vi "Passing Paramters 2D Array Of Integers.vi"(8 "error in (no error)":errorcluster, 9 "cols":i32, 10 "rows":i32, 11 "x":i32) -> (0 "error out":errorcluster, 2 "function return":i32, 3 "x out":i32)   [LabVIEW 2009, in "LabVIEWWrapper_PassingDataSampleDLL.lvlib"]
doc: "int PassingParamters_2DArrayOfIntegers (int *x, int rows, int cols);"
uses:
  LabVIEWWrapper_PassingDataSampleDLL.lvlib
  PassingDataSampleDLL.dll
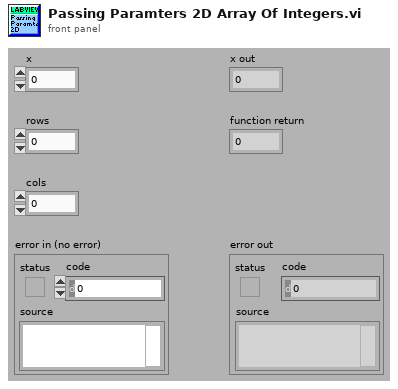
[diagram p1: front panel]
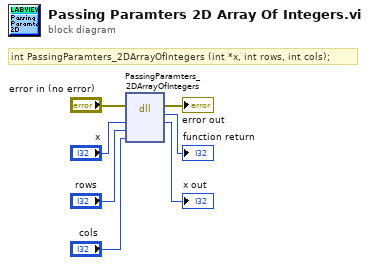
[diagram p0: block diagram]
diagram:
  # "int PassingParamters_2DArrayOfIntegers (int *x, int rows, int cols);"
  n1 = dll-call lib="C:/My Dropbox/Systems Engineering Application/SDK/C Integration/LabVIEWWrapper/PassingDataSampleDLL.*" fn="PassingParamters_2DArrayOfIntegers"(error in="error in (no error)", "x"="x", "rows"="rows", "cols"="cols") -> (error out=→"error out":errorcluster, →"function return":i32, "x"=→"x out":i32)  [unwired: 4 in, 1 out]
